vi "iRobot UART Byte Array Checksum.vi"(1 "Number of Values (-1)":i32=-1, 3 "Byte Array":u8[](array[numeric]) format="%02x") -> (0 "Checksum":u8 format="%02x")   [LabVIEW 2014]
doc: "Returns the sum of the first <b>Number of Values</b> in a byte array."
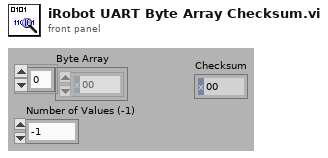
[diagram p1: front panel]
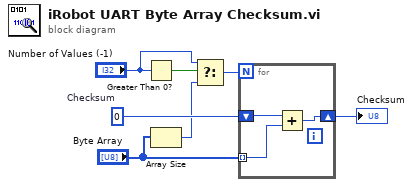
[diagram p0: block diagram]
diagram:
  w7 = u8 0  # Checksum
  n1 = Greater Than 0?(x="Number of Values (-1)") -> (x > 0?=w5:bool)
  n2 = Array Size(array="Byte Array") -> (size(s)=w2:i32)
  n3 = Select(t="Number of Values (-1)", s=w5, f=w2) -> (s? t:f=w1:i32)
  n4 = for {
    N: w1 -> [_]
    tunnel: "Byte Array" -> [w9] mode=indexing
    shift-right: [w8] -> w6
    shift-left: w7 -> [w10]
    n5 = Add(x=w10, y=w9) -> (x+y=w8:u8)
  }
  "Checksum" <- w6
